vi "close_iteration_data_files.vi"(8 "error in (no error)":errorcluster, 9 "Hamamatsu_C9100-13 (in)":refnum<class "Hamamatsu_C9100-13.lvclass">, 10 "Counter (in)":refnum<class "Counter.lvclass">, 11 "ExperimentVariables in":refnum<class "ExperimentVariables.lvclass">) -> (0 "error out":errorcluster, 1 "Hamamatsu_C9100-13":refnum<class "Hamamatsu_C9100-13.lvclass">, 2 "Counter out":refnum<class "Counter.lvclass">, 3 "ExperimentVariables out":refnum<class "ExperimentVariables.lvclass">)   [LabVIEW 2013]
uses:
  Counter/Counter.lvclass
  Camera/Hamamatsu_C9100-13/Hamamatsu_C9100-13.lvclass
  ExperimentVariables.lvclass
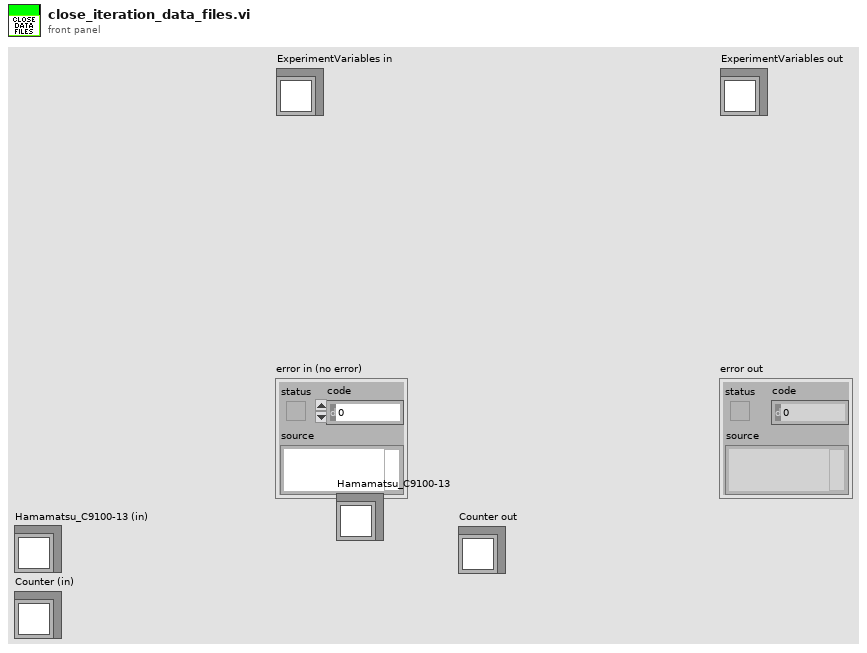
[diagram p1: front panel]
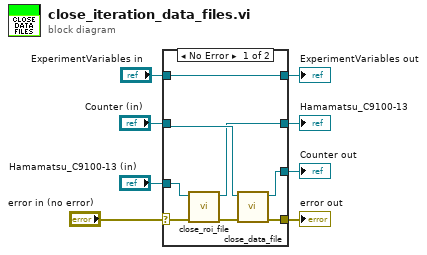
[diagram p0: block diagram]
diagram:
  n1 = case shown="No Error" "error in (no error)" {
    selector: "error in (no error)" -> [w10 w20]
    tunnel: [w9 w20] -> w7
    tunnel: [w16 w19] -> w5
    tunnel: "ExperimentVariables in" -> [w16 w19]
    tunnel: "Counter (in)" -> [w15 w18]
    tunnel: [w14 w18] -> w3
    tunnel: "Hamamatsu_C9100-13 (in)" -> [w13 w17]
    tunnel: [w12 w17] -> w1
    frame No Error {
      n2 = call-dynamic "close_roi_file.vi"("error in (no error)"=w10, "Camera in"=w13) -> ("error out"=w11:errorcluster, "Camera out"=w12:refnum<class "Hamamatsu_C9100-13.lvclass">)  [unwired: 8 in]
      n3 = call-dynamic "close_data_file.vi"("error in (no error)"=w11, "Counter in"=w15) -> ("error out"=w9:errorcluster, "Counter out"=w14:refnum<class "Counter.lvclass">)  [unwired: 8 in]
    }
    frame Error {
    }
  }
  "error out" <- w7
  "ExperimentVariables out" <- w5
  "Hamamatsu_C9100-13" <- w1
  "Counter out" <- w3
